vi "PicoScope5000aExampleETS.vi"() -> ()   [LabVIEW 2010]
doc: "This example demonstrates how to use the PicoScope Labview library to collect data using ETS mode for the ps5000a API."
uses:
  shared/PicoBuffers.ctl
  PicoScope5000aLib/PicoScope5000aAnalogChannelSettings.ctl
  shared/Buffer and Transfer Settings.ctl
  shared/Acquisition Settings.ctl
panel:
  out "Properties Panel":T1 {"Max Total Capture Time Available (sec)" format="%.3p"; "Sample Frequency" format="%.3p"; "Sample Rate" format="%.3p"; "Max Samples Available" format="%.3p"; "Total Capture Time (sec)" format="%.3p"}
  out "EtsTimeValues":i64[](array[numeric])
  in  "ETS Mode":u32(ring)=1 items=["PS5000A_ETS_OFF", "PS5000A_ETS_FAST", "PS5000A_ETS_SLOW"]
  in  "etsInterleave":i16=20
  in  "etsCycles":i16=100
  out "overflow":i16 format="%010b"
  in  "Apply Settings":bool
  in  "Channel A Settings":T2={"Enabled"=TRUE, "Coupling"=1, "Range"=6, "Analogue Offset"=0.0, "Bandwidth Limit"=0} {"Bandwidth Limit" items=["Full", "20MHz"]; "Range" items=["10 mV", "20 mV", "50 mV", "100 mV", "200 mV", "500 mV", "1 V", "2 V", "5 V", "10 V", "20 V"]; "Coupling" items=["AC", "DC"]}
  in  "Trigger Settings":T3={"Trigger Enabled"=TRUE, "Trigger Source"=enum."Channel A", "Trigger Threshold (volts)"=0.0, "Trigger Direction"=2, "Trigger Delay (samples)"=0, "Auto Trigger Time (ms)"=1000} {"Trigger Direction" items=["Rising"=2, "Falling"=3]}
  out "USB 3.0 device on non-USB 3.0 Port":bool=TRUE
  out "USB Powered":bool=TRUE
  out "Device Info":T4={"Driver Version"="2.1.104.3324", "USB Version"="2.0", "Hardware"="1", "Variant"="5244A", "Batch and Serial"="CQ178/007", "Cal Date"="11Jun13", "Kernel Version"="1.0", "Digital HW Version"="1", "Analogue HW Version"="1", "MSO"=FALSE, "Number of channels"=2}
  out "error out":errorcluster
  in  "Data file":path=path "PicoScope5000aExampleETS ChA Data"
  in  "Buffer and Transfer Settings":T5={"startIndex"=0, "Samples"=1000, "Down Sample Ratio"=1, "Down-Sample Mode"=0} {"Down-Sample Mode" items=["RAW none"=2147483648, "None"=0, "Aggregate"=1, "Decimate"=2, "Average"=4]; "Down Sample Ratio" step=1; "Samples" format="%_6p"}
  in  "Acquisition Settings":T6={"preTriggerSamples"=0, "postTriggerSamples"=1000, "timebase"=0} {"postTriggerSamples" format="%_6p"; "preTriggerSamples" format="%_6p"}
  in  "stop":bool
  out "Analog Channels":cluster{i32, sgl, "Data":dbl[]}(graph)
  in  "Serial Number":string
  in  "Use Serial Number":bool
  in  "error in (no error)":errorcluster
  # "ETS mode - NOTE is only on Channel A at 8-bit ADC resolution"
  # "Maximum values are based on model number"
  # "Bit 0 = ChA"
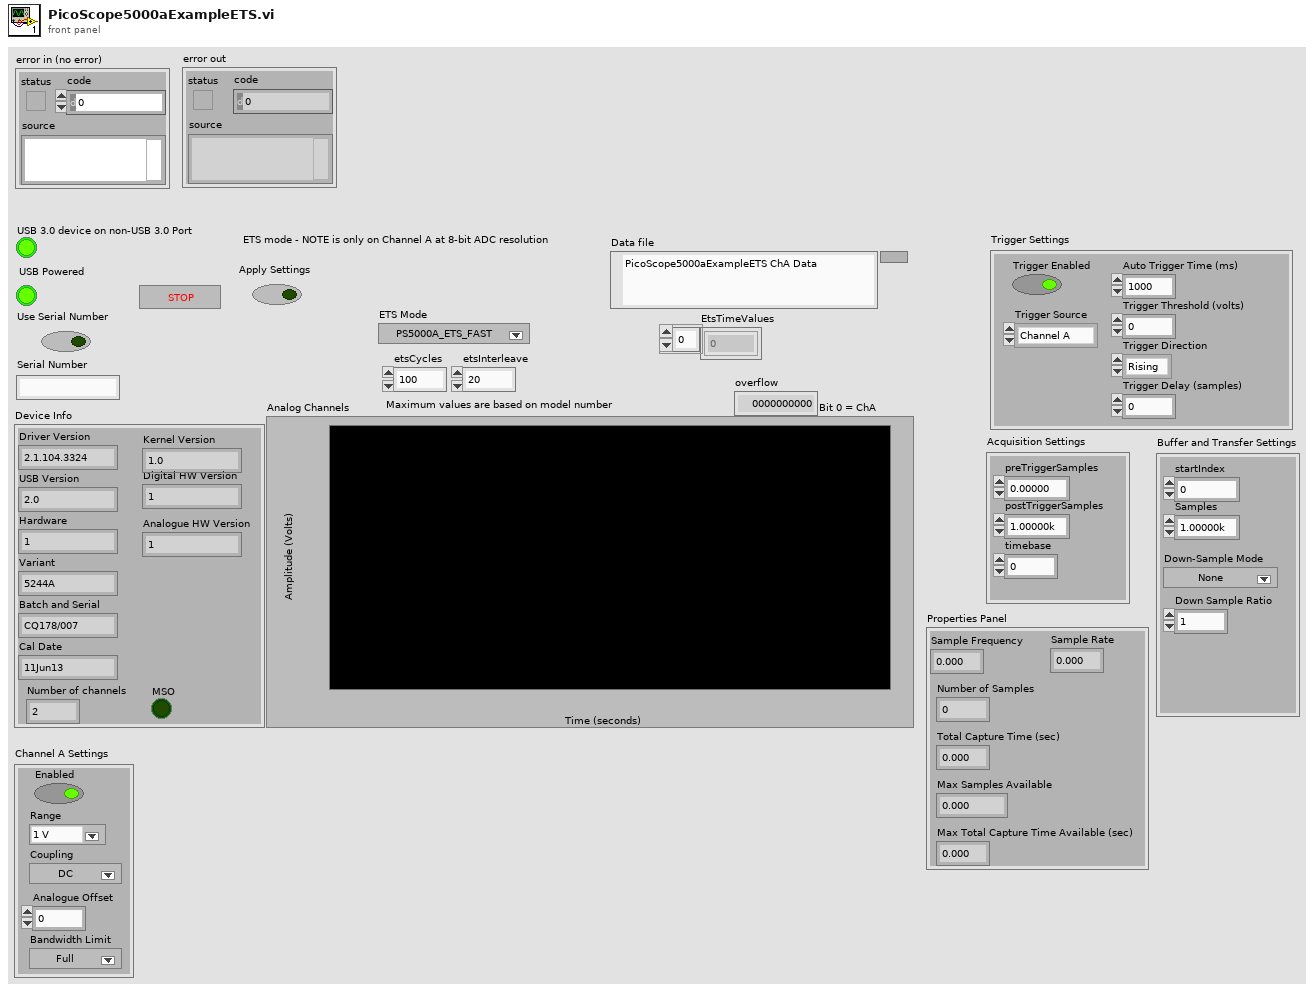
[diagram p1: front panel]
types:
  T1 = cluster{"Sample Frequency":sgl, "Sample Rate":sgl, "Max Samples Available":i32, "Number of Samples":u32, "Total Capture Time (sec) ":sgl, "Max Total Capture Time Available (sec)":sgl}
  T2 = typedef "PicoScope5000aAnalogChannelSettings.ctl" = cluster{"Enabled":bool, "Coupling":i16, "Range":u16, "Analogue Offset":sgl, "Bandwidth Limit":u32}
  T3 = cluster{"Trigger Enabled":bool, "Trigger Source":enum16{"Channel A", "Channel B", "Channel C", "Channel D", "Ext."}, "Trigger Threshold (volts)":dbl, "Trigger Direction":u16, "Trigger Delay (samples)":u32, "Auto Trigger Time (ms)":i16}
  T4 = cluster{"Driver Version":string, "USB Version":string, "Hardware":string, "Variant":string, "Batch and Serial":string, "Cal Date":string, "Kernel Version":string, "Digital HW Version":string, "Analogue HW Version":string, "MSO":bool, "Number of channels":i16}
  T5 = typedef "Buffer and Transfer Settings.ctl" = cluster{"startIndex":u64, "Samples":u64, "Down Sample Ratio":u64, "Down-Sample Mode":u32}
  T6 = typedef "Acquisition Settings.ctl" = cluster{"preTriggerSamples":u64, "postTriggerSamples":u64, "timebase":u32}
  T7 = typedef "PicoBuffers.ctl" = cluster{"Max Buffer Pointers":u64[][][], "Min Buffer Pointers":u64[][][], "StreamingDataInfo":cluster{"Channel":u32, "Down-Sample Mode":u32, "PICO_DATA_TYPE":enum32{"PICO_INT8_T", "PICO_INT16_T", "PICO_INT32_T", "PICO_UINT32_T", "PICO_INT64_T", ""}, "Samples":i32, "bufferIndex":u64, "startIndex":i32, "overflow":i16}[][]}
  T8 = enum16{"open", "open or create", "create or replace", "create", "open (read-only)"}
  T9 = cluster{"Channel A Buffer":i16[], "Channel B Buffer":i16[], "Channel C Buffer":i16[], "Channel D Buffer":i16[], "Channel E Buffer":i16[], "Channel F Buffer":i16[], "Channel G Buffer":i16[], "Channel H Buffer":i16[], "Port 0 Buffer":i16[], "Port 1 Buffer":i16[]}[]
  T10 = cluster{"Channel A Buffer":i16[], "Channel B Buffer":i16[], "Channel C Buffer":i16[], "Channel D Buffer":i16[], "Channel E Buffer":i16[], "Channel F Buffer":i16[], "Channel G Buffer":i16[], "Channel H Buffer":i16[], "Port 0 Buffer":i16[], "Port 1 Buffer":i16[]}
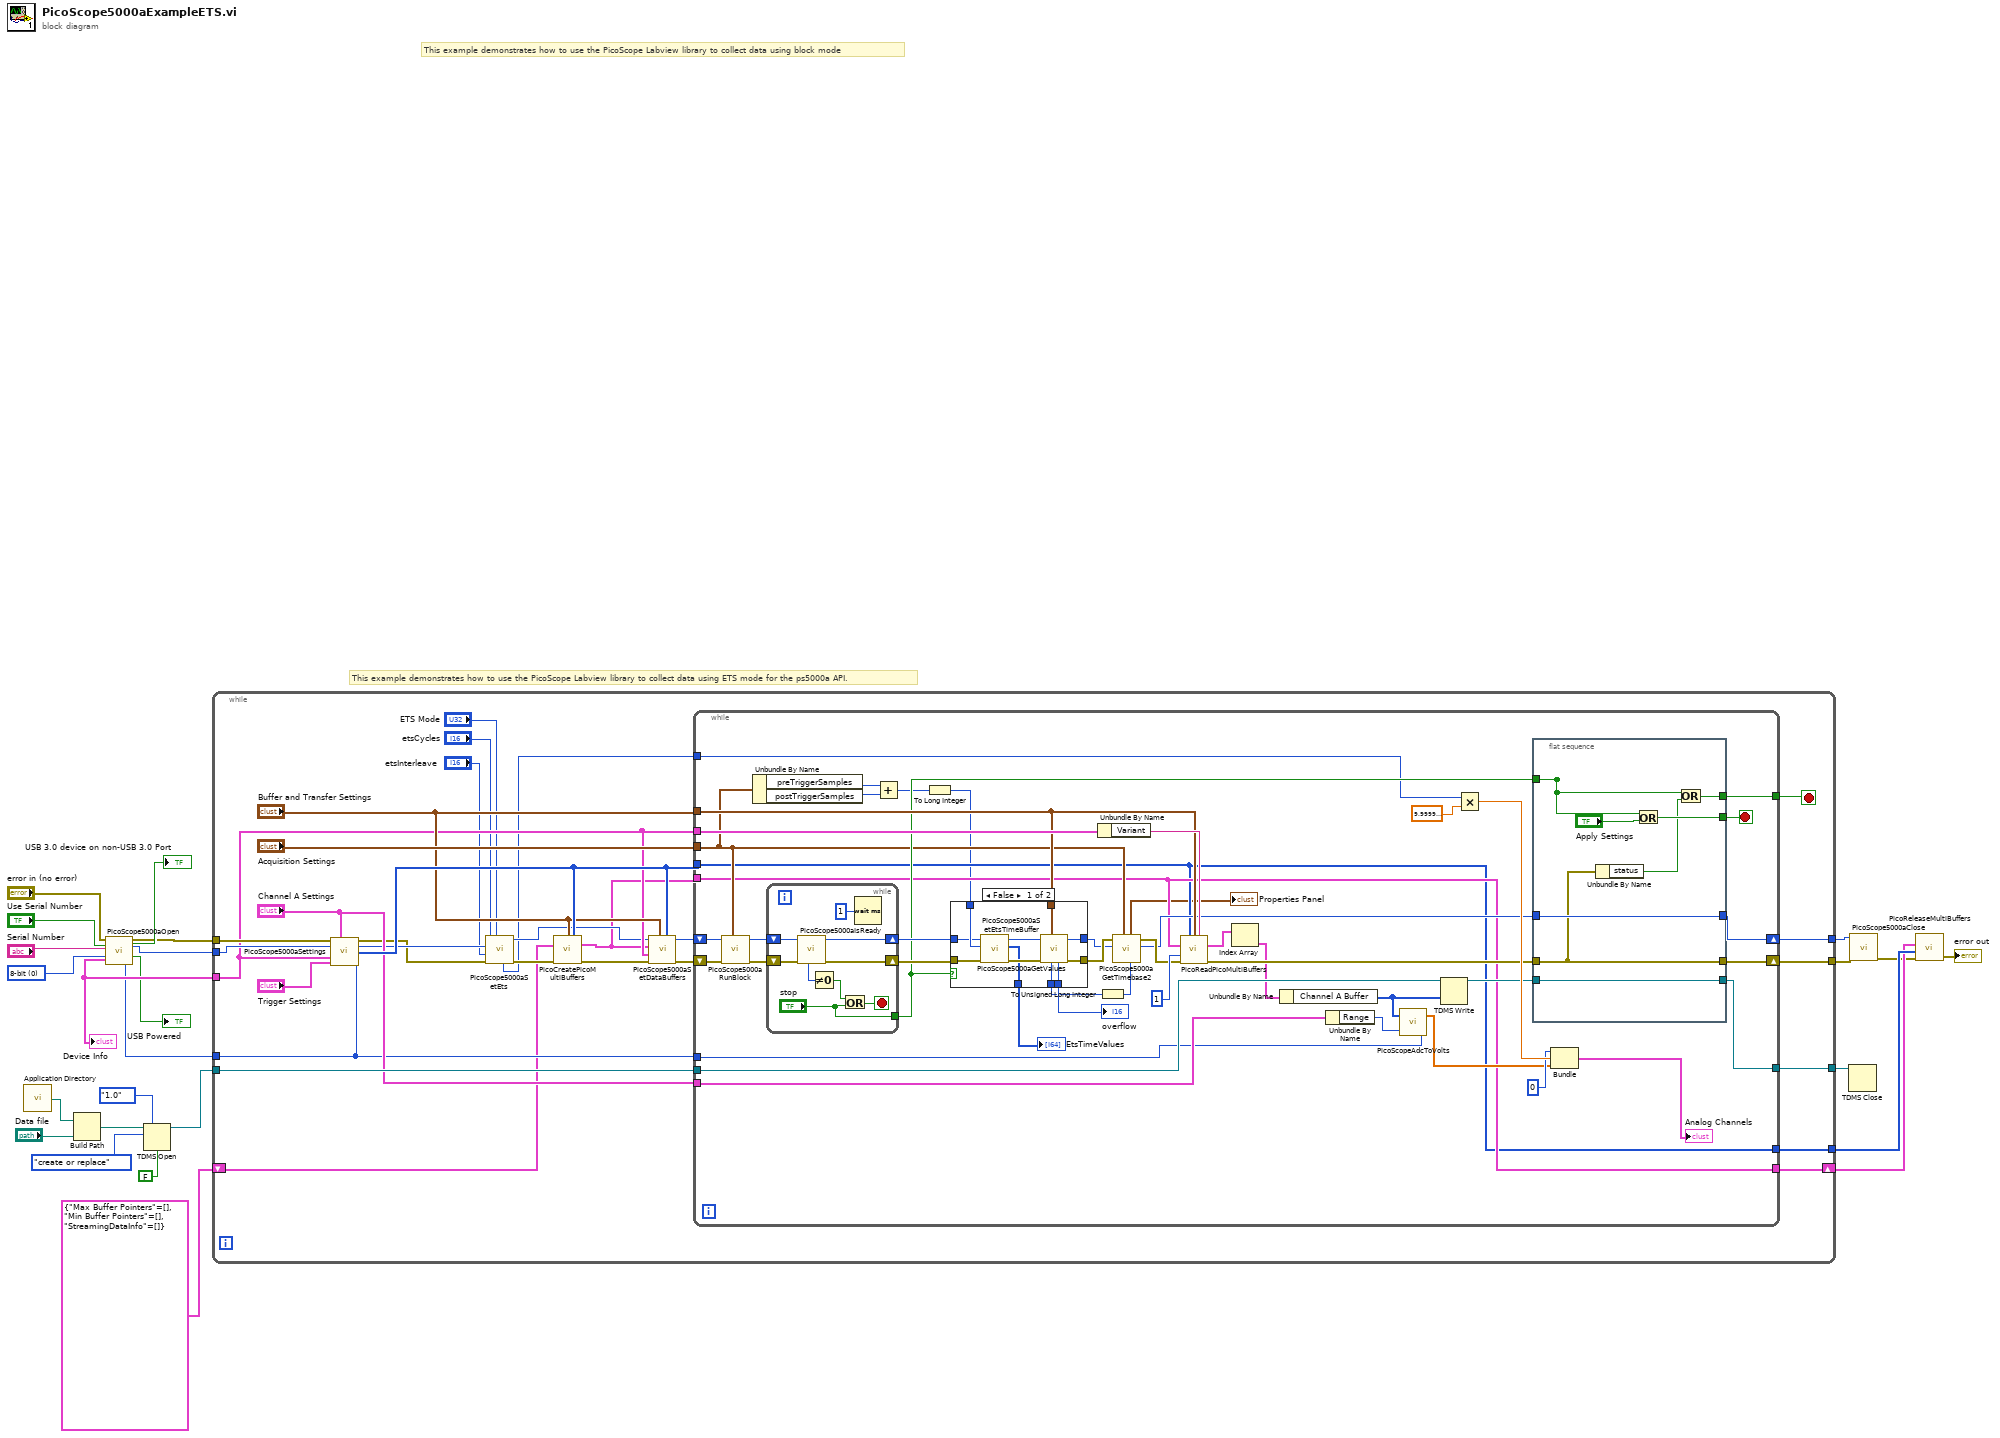
[diagram p0: block diagram]
diagram:
  w12 = u32 0 items=["8-bit"=0, "12-bit"=1, "14-bit"=2, "15-bit"=3, "16-bit"=4, "10-bit"=10] ("Resolution")
  # "This example demonstrates how to use the PicoScope Labview library to collect data using ETS mode for the ps5000a API."
  # "This example demonstrates how to use the PicoScope Labview library to collect data using block mode"
  n1 = call <vilib>:"Application Directory.vi"() -> ("Application Directory"=w17:path)
  n2 = Build Path(base path=w17, name or relative path="Data file") -> (appended path=w18:path)
  n3 = call "PicoScope5000aOpen.vi"("error in (no error)"="error in (no error)", "Serial Number"="Serial Number", "Use Serial Number"="Use Serial Number", "Resolution"=w12) -> ("USB 3.0 device on non-USB 3.0 Port"=→"USB 3.0 device on non-USB 3.0 Port":bool, "error out"=w5:errorcluster, "handle"=w25:i16, "USB Powered"=→"USB Powered":bool, "Device Info"=w9:T4, "Max ADC value"=w8:i16)  [unwired: 6 in]
  "Device Info" <- w9
  n4 = TDMS Open(6:FALSE ("disable buffering? (T)"), 7:enum16{"1.0", "2.0"}."1.0" ("file format version (2.0)"), 10:T8."create or replace" ("operation (0:open)"), 11:w18) -> (3:w15:refnum<k34>)  [unwired: 2 in, 1 out]
  n5 = while {
    tunnel: w25 -> [w52]
    tunnel: w8 -> [w46]
    tunnel: [w27] -> w24
    tunnel: [w45] -> w16
    tunnel: w15 -> [w53]
    tunnel: w9 -> [w39]
    tunnel: w5 -> [w51]
    tunnel: [w43] -> w4
    shift-right: [w28] -> w23
    shift-left: T7 {"Max Buffer Pointers"=[], "Min Buffer Pointers"=[], "StreamingDataInfo"=[]} ("Data Pointers") -> [w30]
    tunnel: [w26] -> w2
    stop <- w44 stop-if-true
    n6 = call "PicoScope5000aSettings.vi"("error in"=w51, "Channel A Settings"="Channel A Settings", "handle in"=w52, "Device Info"=w39, "Trigger Settings"="Trigger Settings", "Max ADC value"=w46) -> ("error out"=w35:errorcluster, "handle out"=w36:i16, "enabled array"=w49:i16[])  [unwired: 7 in]
    n7 = call "PicoScope5000aSetEts.vi"("ETS Mode"="ETS Mode", "error in (no error)"=w35, "etsInterleave"="etsInterleave", "etsCycles"="etsCycles", "handle in"=w36) -> ("error out"=w38:errorcluster, "handle out"=w37:i16, "sampleTimePicoseconds"=w31:i32)  [unwired: 4 in]
    n8 = call "PicoCreatePicoMultiBuffers.vi"("Buffer and Transfer Settings"="Buffer and Transfer Settings", "enabled array"=w49, "Data Pointers In"=w30, "error in (no error)"=w38) -> ("Data Pointers"=w29:T7, "error out"=w54:errorcluster)  [unwired: 10 in]
    n9 = call "PicoScope5000aSetDataBuffers.vi"("enabled array"=w49, "Buffer and Transfer Settings"="Buffer and Transfer Settings", "error in (no error)"=w54, "Device Info"=w39, "Data Pointers In"=w29, "handle in"=w37) -> ("error out"=w42:errorcluster, "handle out"=w41:i16)  [unwired: 4 in]
    n10 = while {
      tunnel: w29 -> [w59]
      tunnel: "Buffer and Transfer Settings" -> [w76]
      tunnel: w49 -> [w58]
      tunnel: "Channel A Settings" -> [w96]
      tunnel: "Acquisition Settings" -> [w62]
      tunnel: w46 -> [w95]
      tunnel: w39 -> [w93]
      tunnel: [w83] -> w44
      shift-right: [w87] -> w26
      shift-left: w42 -> [w77]
      shift-right: [w81] -> w43
      shift-left: w41 -> [w78]
      tunnel: w53 -> [w101]
      tunnel: [w85] -> w45
      tunnel: w31 -> [w65]
      tunnel: [w59] -> w28
      tunnel: [w58] -> w27
      stop <- w82 stop-if-true
      n11 = call "PicoScope5000aRunBlock.vi"("Acquisition Settings"=w62, "error in (no error)"=w77, "handle in"=w78) -> ("error out"=w98:errorcluster, "handle out"=w97:i16)  [unwired: 5 in, 2 out]
      n12 = Unbundle By Name(w62) -> ("preTriggerSamples"=w64:u64, "postTriggerSamples"=w63:u64)
      n13 = while {
        shift-right: [w130] -> w79
        shift-left: w98 -> [w131]
        shift-right: [w129] -> w80
        shift-left: w97 -> [w128]
        tunnel: ["stop"] -> w75
        stop <- w125 stop-if-true
        n14 = call "PicoScope5000aIsReady.vi"("error in (no error)"=w131, "handle in"=w128) -> ("error out"=w130:errorcluster, "handle out"=w129:i16, "ready"=w127:i16)  [unwired: 7 in]
        n15 = Not Equal To 0?(x=w127) -> (x != 0?=w126:bool)
        n16 = Or(x=w126, y="stop") -> (x .or. y?=w125:bool)
        n17 = Wait (ms)(milliseconds to wait=u32 1) -> ()  [unwired: 1 out]
      }
      n18 = Add(x=w64, y=w63) -> (x+y=w56:u64)
      n19 = To Long Integer(number=w56) -> (32bit integer=w55:i32)
      n20 = case shown="False" w75 {
        tunnel: w79 -> [w105 w113]
        tunnel: w80 -> [w106 w114]
        tunnel: [w112 w114] -> w72
        tunnel: [w111 w113] -> w73
        tunnel: w76 -> [w110 _]
        tunnel: [w109 _] -> w74
        tunnel: [w108 _] -> w69
        tunnel: w55 -> [w107 _]
        tunnel: [w102 _] -> w61
        frame False {
          n21 = call "PicoScope5000aSetEtsTimeBuffer.vi"("error in (no error)"=w105, "bufferLth"=w107, "handle in"=w106) -> ("error out"=w104:errorcluster, "EtsTimeValues"=w102:i64[], "handle out"=w103:i16)  [unwired: 6 in]
          n22 = call "PicoScope5000aGetValues.vi"("Buffer and Transfer Settings"=w110, "error in (no error)"=w104, "handle in"=w103) -> ("error out"=w111:errorcluster, "handle out"=w112:i16, "overflow"=w109:i16, "noOfSamples"=w108:u64)  [unwired: 5 in]
        }
        frame True {
        }
      }
      "overflow" <- w74
      "EtsTimeValues" <- w61
      n23 = Unbundle By Name(w93) -> ("Variant"=w94:string)
      n24 = To Unsigned Long Integer(number=w69) -> (unsigned 32bit integer=w68:u32)
      n25 = call "PicoScope5000aGetTimebase2.vi"("Number of Samples"=w68, "Acquisition Settings"=w62, "handle in"=w72, "error in (no error)"=w73) -> ("handle out"=w70:i16, "error out"=w71:errorcluster, "Properties Panel"=→"Properties Panel":T1)  [unwired: 5 in]
      n26 = call "PicoReadPicoMultiBuffers.vi"("enabled array"=w58, "Buffer and Transfer Settings"=w76, "Variant"=w94, "Data Pointers"=w59, "No of Buffers"=1, "error in (no error)"=w71) -> ("MultiBuffers (Max or non-aggregated)"=w100:T9, "error out"=w84:errorcluster)  [unwired: 7 in, 1 out]
      n27 = Index Array(array=w100) -> (element=w66:T10)  [unwired: 1 in]
      n28 = Unbundle By Name(w66) -> ("Channel A Buffer"=w88:i16[])
      n29 = Unbundle By Name(w96) -> ("Range"=w90:u16)
      n30 = call "PicoScopeAdcToVolts.vi"("Max_adc"=w95, "Range Index"=w90, "Data"=w88) -> ("Data"=w89:dbl[])
      n31 = TDMS Write(0:w101, 9:w88) -> (4:w86:refnum<k34>)  [unwired: 4 in, 3 out]
      n32 = Multiply(x=w65, y=sgl 1e-12) -> (x*y=w99:sgl)
      n33 = flat-sequence {
        tunnel: [w122] -> w82
        tunnel: [w115] -> _
        tunnel: [w119] -> w83
        tunnel: w70 -> [w118]
        tunnel: [w118] -> w81
        tunnel: w84 -> [w117]
        tunnel: [w117] -> w87
        tunnel: [w116] -> w85
        tunnel: w86 -> [w116]
        tunnel: w75 -> [w115]
        frame #0 {
          n34 = Unbundle By Name(w117) -> ("status"=w120:bool)
          n35 = Or(x=w115, y="Apply Settings") -> (x .or. y?=w122:bool)
          n36 = Or(x=w115, y=w120) -> (x .or. y?=w119:bool)
        }
      }
      n37 = Bundle(0, w99, "Data"=w89) -> (→"Analog Channels":cluster{i32, sgl, "Data":dbl[]})  [unwired: 1 in]
    }
  }
  n38 = TDMS Close(11:w16) -> ()  [unwired: 1 in, 2 out]
  n39 = call "PicoScope5000aClose.vi"("error in (no error)"=w2, "handle in"=w4) -> ("error out"=w1:errorcluster)  [unwired: 8 in, 1 out]
  n40 = call "PicoReleaseMultiBuffers.vi"("error in (no error)"=w1, "Enabled array"=w24, "Data Pointers"=w23) -> ("error out"=→"error out":errorcluster)  [unwired: 7 in, 1 out]
